vi "Configure User-Defined Descriptions.vi"(8 "Error In":errorcluster, 11 "User-Defined Descriptions":string[](array[string])) -> (0 "Error Out":errorcluster)   [LabVIEW 2018, in "Toolkit.lvlib"]
doc: "Adds user-defined descriptions for errors."
uses:
  Toolkit.lvlib
  Support/Error/Error Action.ctl
  Support/Error/Error.lvlib
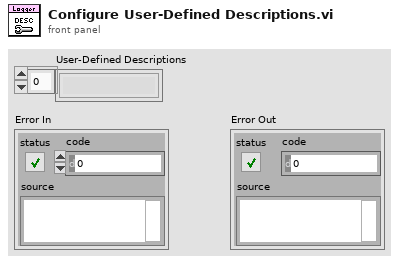
[diagram p1: front panel]
types:
  T1 = typedef "Toolkit.lvlib/Error.lvlib/Error Action.ctl" = enum16{"Initialize", "Get", "Set Verbosity", "Set User-Defined Codes", "Set User-Defined Descriptions", "Shutdown"}
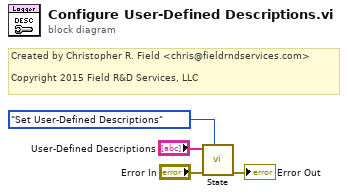
[diagram p0: block diagram]
diagram:
  # "Created by Christopher R. Field <chris@fieldrndservices.com>\n\nCopyright 2015 Field R&D Services, LLC"
  n1 = call "State.vi"("Action"=Error_Action."Set User-Defined Descriptions", "Error In"="Error In", "Set Value"="User-Defined Descriptions") -> ("Error Out"=→"Error Out":errorcluster)  [unwired: 7 in, 1 out]
